vi "Bundle Script_In Place Remove.vi"(8 "error in":errorcluster, 9 "Selected Item Indices":u32[](array[numeric]), 10 "Selected Items Tags":string[](array[string]), 11 "Affected Items":T1) -> (0 "error out":errorcluster)   [LabVIEW 2023]
doc: "Remove elements from In Place cluster bundler."
uses:
  top/BundleMagic.ctl
panel:
  # "OR"
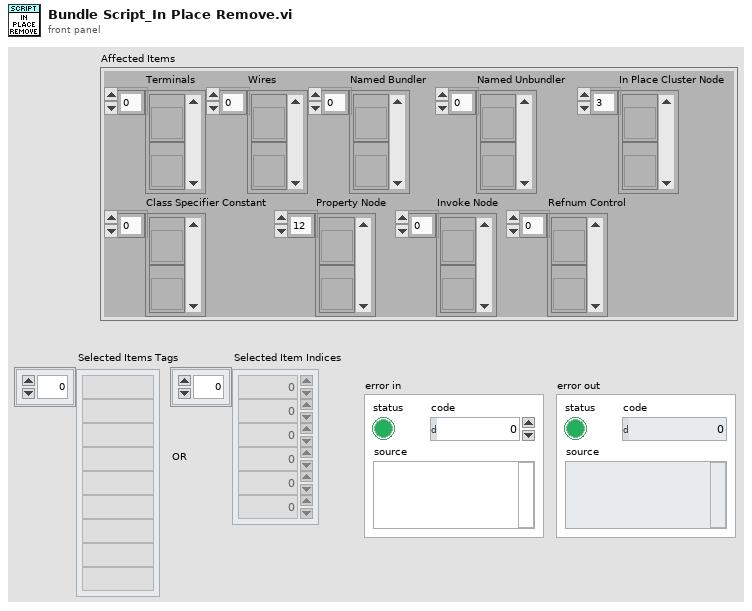
[diagram p1: front panel]
types:
  T1 = typedef "BundleMagic.ctl" = cluster{"Terminals":refnum<vi>[], "Wires":refnum<vi>[], "Named Bundler":refnum<vi>[], "Named Unbundler":refnum<vi>[], "In Place Cluster Node":refnum<vi>[], "Class Specifier Constant":refnum<vi>[], "Property Node":refnum<vi>[], "Invoke Node":refnum<vi>[], "Refnum Control":refnum<vi>[]}
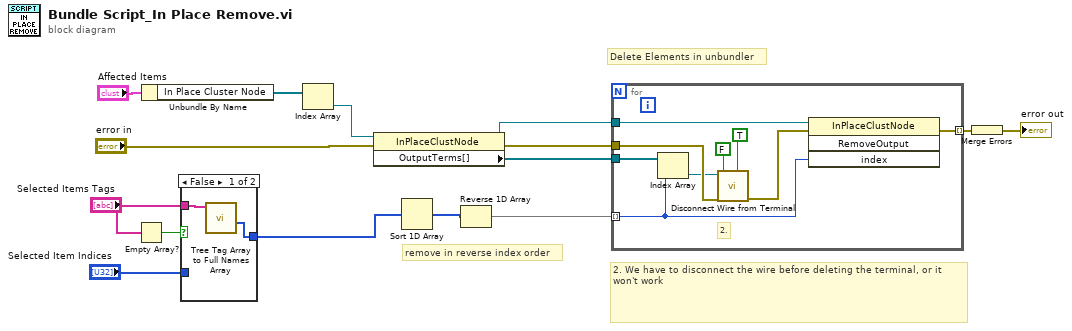
[diagram p0: block diagram]
diagram:
  # "remove in reverse index order"
  # "2. We have to disconnect the wire before deleting the terminal, or it won't work"
  # "Delete Elements in unbundler"
  n1 = Empty Array?(array="Selected Items Tags") -> (empty?=w2:bool)
  n2 = Unbundle By Name("Affected Items") -> ("In Place Cluster Node"=w14:refnum<vi>[])
  n3 = case shown="False" w2 {
    tunnel: "Selected Items Tags" -> [w17 _]
    tunnel: [w16 w18] -> w5
    tunnel: "Selected Item Indices" -> [_ w18]
    frame False {
      n4 = call "Tree Tag Array to Full Names Array.vi"("Selected Items Tags"=w17) -> ("Selected Item Indices"=w16:u32[])  [unwired: 6 in, 4 out]
    }
    frame True {
    }
  }
  n5 = Index Array(array=w14) -> (element=w8:refnum<vi>)  [unwired: 1 in]
  n6 = property class="InPlaceClustNode"(reference=w8, error in="error in") -> (reference out=w10:refnum<vi>, error out=w9:errorcluster, "OutputTerms[]"=w6:refnum<vi>[])
  n7 = Sort 1D Array(array=w5) -> (sorted array=w12:u32[])
  n8 = Reverse 1D Array(array=w12) -> (reversed array=w11:u32[])
  n9 = for {
    tunnel: [w27] -> w13 mode=indexing
    tunnel: w11 -> [w25] mode=indexing
    tunnel: w10 -> [w26]
    tunnel: w9 -> [w21]
    tunnel: w6 -> [w24]
    # "2."
    n10 = Index Array(array=w24, index=w25) -> (element=w20:refnum<vi>)
    n11 = call "Disconnect Wire from Terminal.vi"("Remove Loose Ends"=TRUE, "Clean Up wire"=FALSE ("Remove Loose Ends"), "error in"=w21, "Terminal in"=w20) -> ("error out"=w19:errorcluster)  [unwired: 3 in, 4 out]
    n12 = invoke class="InPlaceClustNode" method="RemoveOutput"(reference=w26, error in=w19, "index"=w25) -> (error out=w27:errorcluster)  [unwired: 1 in, 3 out]
  }
  n13 = Merge Errors(w13) -> (→"error out":errorcluster)
